vi "9. FGV EOT Check.vi"(8 "error in (no error)":errorcluster, 11 "VISA resource name":refnum<visa-resource-name>="COM3") -> (0 "error out":errorcluster, 4 "NO EOT?":bool)   [LabVIEW 2014]
uses:
  control/FGV Serial Tasks.ctl
panel:
  in  "Timeout":dbl
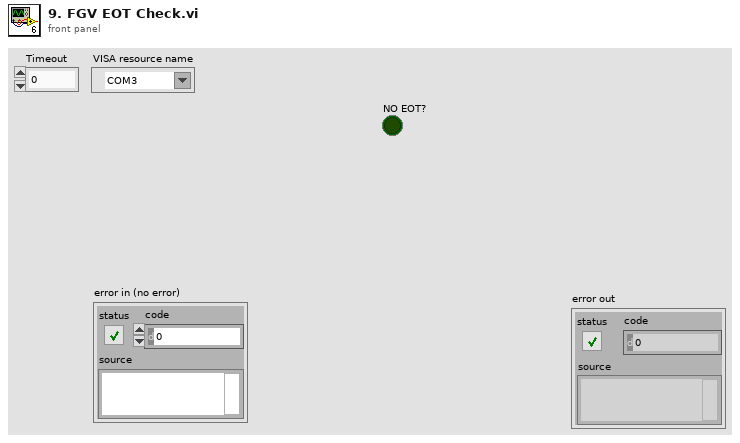
[diagram p1: front panel]
types:
  T1 = typedef "FGV Serial Tasks.ctl" = enum16{"Open", "Read", "Write", "Close", "Flush"}
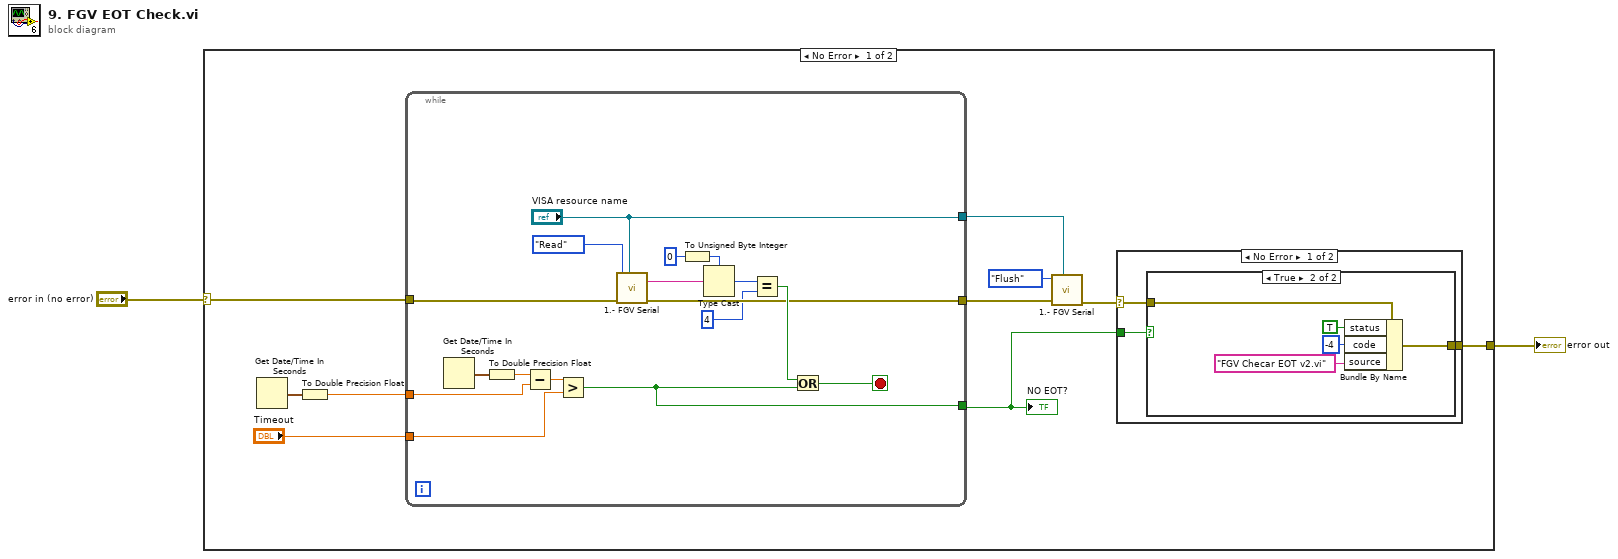
[diagram p0: block diagram]
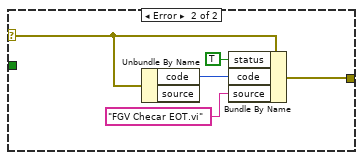
[diagram p3: hidden frame]
diagram:
  n1 = case shown="No Error" "error in (no error)" {
    selector: "error in (no error)" -> [w12 w44]
    tunnel: [w8 w44] -> w1
    frame No Error {
      n2 = Get Date/Time In Seconds() -> (seconds since 1Jan1904=w11:timestamp)
      n3 = To Double Precision Float(number=w11) -> (double precision float=w10:dbl)
      n4 = while {
        tunnel: w12 -> [w43]
        tunnel: w10 -> [w42]
        tunnel: "Timeout" -> [w41]
        tunnel: [w38] -> w7
        tunnel: [w37] -> w4
        tunnel: ["VISA resource name"] -> w3
        stop <- w40 stop-if-true
        n5 = Get Date/Time In Seconds() -> (seconds since 1Jan1904=w35:timestamp)
        n6 = To Double Precision Float(number=w35) -> (double precision float=w34:dbl)
        n7 = Subtract(x=w34, y=w42) -> (x-y=w33:dbl)
        n8 = Greater?(x=w33, y=w41) -> (0:w38:bool)
        n9 = call "1.- FGV Serial.vi"("VISA resource name"="VISA resource name", "error in (no error)"=w43, "Task"=FGV_Serial_Tasks."Read") -> ("error out"=w37:errorcluster, "Receive buffer"=w31:string)  [unwired: 6 in, 1 out]
        n10 = To Unsigned Byte Integer(number=u8 0) -> (unsigned 8bit integer=w30:u8)
        n11 = Type Cast(type=w30, x=w31) -> (*(type *) &x=w28:u8)
        n12 = Equal?(x=w28, y=u8 4) -> (x = y?=w39:bool)
        n13 = Or(x=w39, y=w38) -> (x .or. y?=w40:bool)
      }
      "NO EOT?" <- w7
      n14 = call "1.- FGV Serial.vi"("VISA resource name"=w3, "error in (no error)"=w4, "Task"=FGV_Serial_Tasks."Flush") -> ("error out"=w5:errorcluster)  [unwired: 6 in, 2 out]
      n15 = case shown="No Error" w5 {
        selector: w5 -> [w13 w22]
        tunnel: [w14 w23] -> w8
        tunnel: w7 -> [w15 _]
        frame No Error {
          n16 = case shown="True" w15 {
            tunnel: [w16 w21] -> w14
            tunnel: w13 -> [w16 w20]
            frame False {
            }
            frame True {
              n17 = Bundle By Name(cluster=w20, "status"=TRUE, "code"=-4, "source"="FGV Checar EOT v2.vi") -> (w21:errorcluster)
            }
          }
        }
        frame Error {
          n18 = Unbundle By Name(w22) -> ("code"=w26:i32)  [unwired: 1 out]
          n19 = Bundle By Name(cluster=w22, "status"=TRUE, "code"=w26, "source"="FGV Checar EOT.vi") -> (w23:errorcluster)
        }
      }
    }
    frame Error {
    }
  }
  "error out" <- w1
